vi "HIOKI PW3390 Initialize.vi"   [LabVIEW 2018]
doc: "Starts the communication with the PW3390 device. This VI can select the communication interface from either LAN or RS-232C."
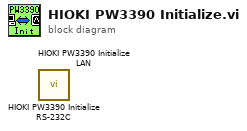
[diagram p0: block diagram]
diagram:
  n1 = call "HIOKI PW3390 Initialize RS-232C.vi"() -> ()  [unwired: 13 in, 3 out]
  n2 = call "HIOKI PW3390 Initialize LAN.vi"() -> ()  [unwired: 13 in, 3 out]
